vi "Build Google Campaign URL.vi"(4 "Campaign Content":string, 6 "Campaign Term":string, 7 "Campaign Medium":string, 8 "Error In":errorcluster, 9 "Campaign Source":string, 10 "Campaign Name":string, 11 "URL":string) -> (0 "Error Out":errorcluster, 3 "Campaign URL":string)   [LabVIEW 2014, in "LMH-Toolbox.lvlib"]
uses:
  <vilib>/MakerHub/Toolbox/LMH-Toolbox.lvlib
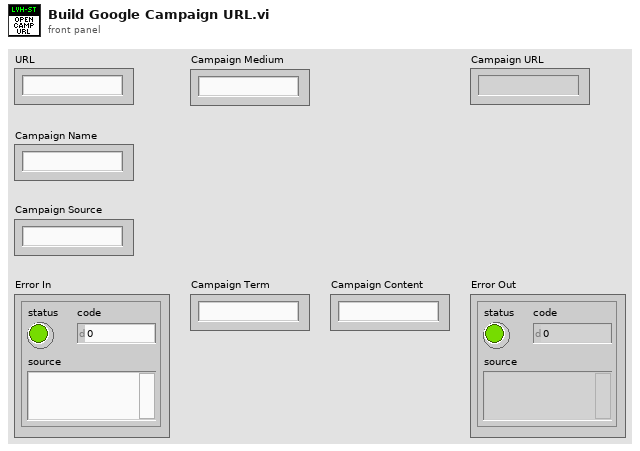
[diagram p1: front panel]
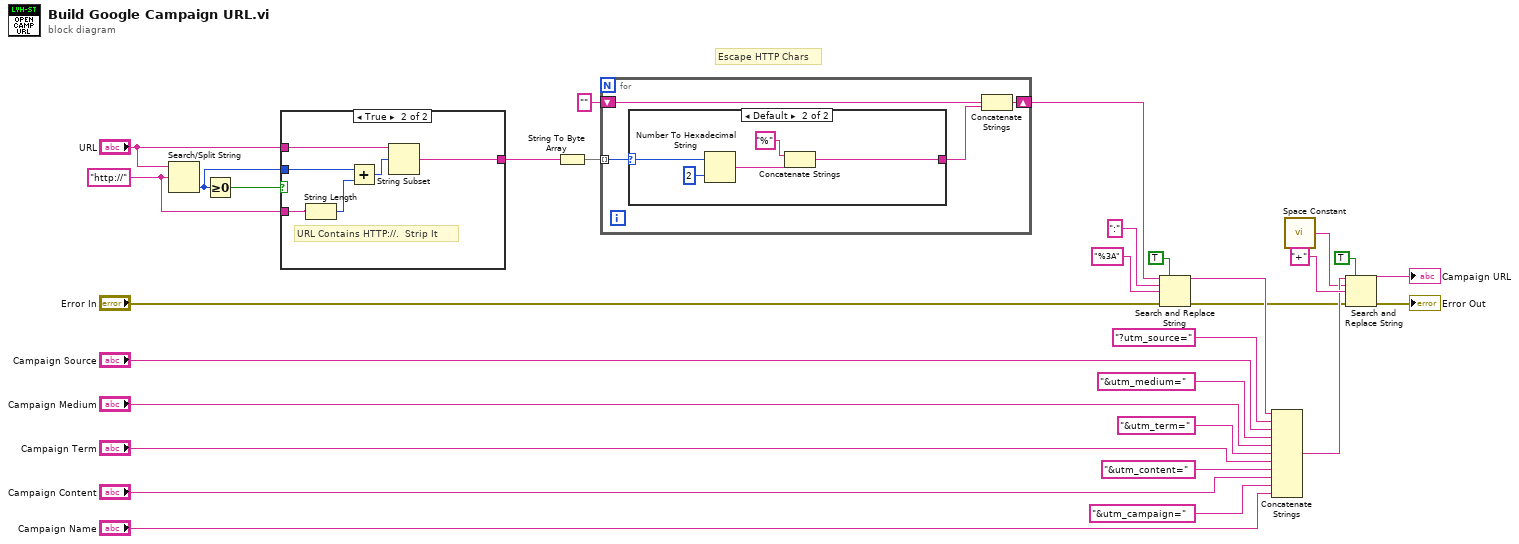
[diagram p0: block diagram]
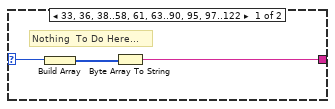
[diagram p2: hidden frame]
diagram:
  w5 = "http://" ("regular expression")
  # "Escape HTTP Chars"
  n1 = Search/Split String(string="URL", search string/char (-)=w5) -> (offset of match=w7:i32)  [unwired: 1 in, 2 out]
  n2 = Greater Or Equal To 0?(x=w7) -> (x >= 0?=w8:bool)
  n3 = case shown="True" w8 {
    tunnel: w7 -> [_ w34]
    tunnel: "URL" -> [w31 w37]
    tunnel: w5 -> [_ w36]
    tunnel: [w31 w32] -> w3
    frame False {
      # "URL Does Not Contain HTTP://\nUse Entire URL"
    }
    frame True {
      # "URL Contains HTTP://.  Strip It"
      n4 = String Length(string=w36) -> (length=w35:i32)
      n5 = Add(x=w34, y=w35) -> (x+y=w33:i32)
      n6 = String Subset(string=w37, offset (0)=w33) -> (substring=w32:string)  [unwired: 1 in]
    }
  }
  n7 = String To Byte Array(string=w3) -> (unsigned byte array=w4:u8[])
  n8 = for {
    shift-right: [w38] -> w2
    shift-left: "" -> [w39]
    tunnel: w4 -> [w41] mode=indexing
    n9 = case shown="Default" w41 {
      selector: w41 -> [w44 w47]
      tunnel: [w42 w46] -> w40
      frame 33, 36, 38..58, 61, 63..90, 95, 97..122 {
        # "Nothing  To Do Here..."
        n10 = Build Array(w44) -> (w43:u8[])
        n11 = Byte Array To String(unsigned byte array=w43) -> (string=w42:string)
      }
      frame Default {
        n12 = Number To Hexadecimal String(1:i16 2 ("width (-)"), 2:w47) -> (0:w48:string)
        n13 = Concatenate Strings("%" ("string"), w48) -> (w46:string)
      }
    }
    n14 = Concatenate Strings(w39, w40) -> (w38:string)
  }
  n15 = Search and Replace String(replace all?=TRUE ("replace all? (F)"), input string=w2, search string=":", replace string="%3A" ("replace string (\"\")"), error in="Error In") -> (result string=w26:string, error out=w12:errorcluster)  [unwired: 3 in, 2 out]
  n16 = Concatenate Strings(w26, "?utm_source=" ("string"), "Campaign Source", "&utm_medium=" ("string"), "Campaign Medium", "&utm_term=" ("string"), "Campaign Term", "&utm_content=" ("string"), "Campaign Content", "&utm_campaign=" ("string"), "Campaign Name") -> (w13:string)
  n17 = call <vilib>:"Space Constant.vi"() -> ("String"=w9:string)
  n18 = Search and Replace String(replace all?=TRUE ("replace all? (F)"), input string=w13, search string=w9, replace string="+" ("replace string (\"\")"), error in=w12) -> (result string=→"Campaign URL":string, error out=→"Error Out":errorcluster)  [unwired: 3 in, 2 out]
